vi "Write InitialState to top file.vi"(8 "error in (no error)":errorcluster, 10 "InitialState":T2, 11 "Refnum in":T1) -> (0 "error out":errorcluster, 3 "Refnum out":T1)   [LabVIEW 2015, in "SLSC Switch.lvlib" / "SLSC Switch.lvclass"]
uses:
  SLSC Switch.lvclass
  Controls/JSON.InitialState.ctl
  <vilib>/Utility/config.llb/Config Data RefNum.ctl
  <vilib>/Utility/config.llb/NI_LVConfig.lvlib
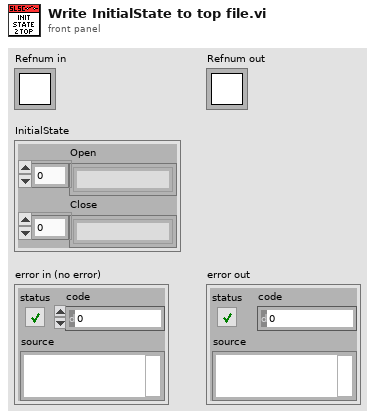
[diagram p1: front panel]
types:
  T1 = typedef "NI_LVConfig.lvlib/Config Data RefNum.ctl" = refnum<k1>
  T2 = typedef "SLSC Switch.lvlib/SLSC Switch.lvclass/JSON.InitialState.ctl" = cluster{"Open":string[], "Close":string[]}
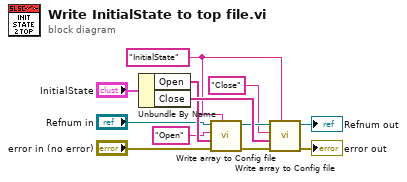
[diagram p0: block diagram]
diagram:
  w7 = "InitialState" ("section")
  n1 = Unbundle By Name("InitialState") -> ("Open"=w11:string[], "Close"=w12:string[])
  n2 = call "Write array to Config file.vi"("section"=w7, "error in (no error)"="error in (no error)", "Array"=w11, "key"="Open", "Refnum in"="Refnum in") -> ("error out"=w2:errorcluster, "refnum out"=w6:T1)  [unwired: 5 in]
  n3 = call "Write array to Config file.vi"("section"=w7, "error in (no error)"=w2, "Array"=w12, "key"="Close", "Refnum in"=w6) -> ("error out"=→"error out":errorcluster, "refnum out"=→"Refnum out":T1)  [unwired: 5 in]
